vi "Overlay Landmark.vi"(6 "Color":u32(colorbox)=16711680, 7 "Group":string, 8 "error in":errorcluster, 9 "Bounding Box":cluster{"x":dbl, "y":dbl}[](array[cluster]), 10 "Position":cluster{"x":sgl, "y":sgl}, 11 "Image":T1) -> (0 "error out":errorcluster, 3 "Image Out":T1)   [LabVIEW 2024]
uses:
  <vilib>/vision/Image Controls.llb/IMAQ Image.ctl
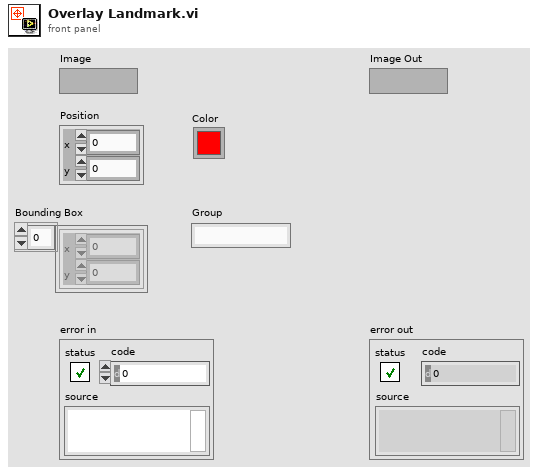
[diagram p1: front panel]
types:
  T1 = typedef "IMAQ Image.ctl" = refnum<image>
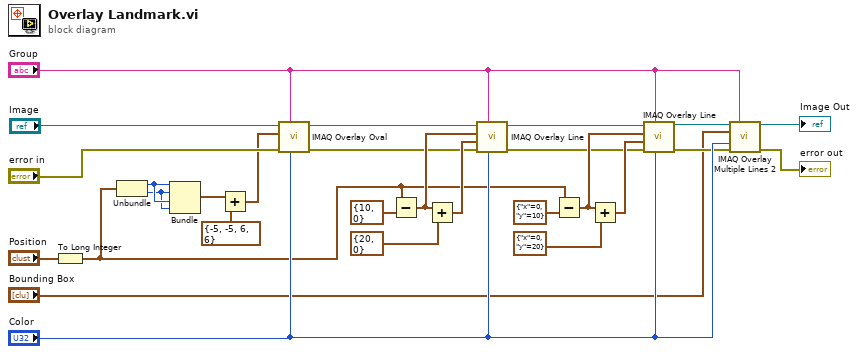
[diagram p0: block diagram]
diagram:
  n1 = To Long Integer(number="Position") -> (32bit integer=w2:cluster{"x":i32, "y":i32})
  n2 = Unbundle(w2) -> ("x"=w20:i32, "y"=w19:i32)
  n3 = Bundle("x"=w20, "y"=w19, "x"=w20, "y"=w19) -> (w18:cluster{"x":i32, "y":i32, "x":i32, "y":i32})  [unwired: 1 out]
  n4 = Add(x=w18, y=cluster{"y":i32, "x":i32, "y":i32, "x":i32} {"y"=-5, "x"=-5, "y"=6, "x"=6}) -> (x+y=w16:cluster{i32, i32, i32, i32})
  n5 = call "IMAQ Overlay Oval"("Color"="Color", "Group"="Group", "error in (no error)"="error in", "Bounding Rectangle"=w16, "Image"="Image") -> ("error out"=w6:errorcluster, "Image Out"=w22:T1)  [unwired: 1 in, 4 out]
  n6 = Subtract(x=w2, y=cluster{"x":i32, "y":i32} {"x"=10, "y"=0}) -> (x-y=w14:cluster{"x":i32, "y":i32})
  n7 = Add(x=w14, y=cluster{"x":i32, "y":i32} {"x"=20, "y"=0}) -> (x+y=w12:cluster{"x":i32, "y":i32})
  n8 = call "IMAQ Overlay Line"("Color"="Color", "Group"="Group", "error in (no error)"=w6, "End Point"=w12, "Start Point"=w14, "Image"=w22) -> ("error out"=w5:errorcluster, "Image Out"=w7:T1)  [unwired: 4 out]
  n9 = Subtract(x=w2, y=cluster{"x":i32, "y":i32} {"x"=0, "y"=10}) -> (x-y=w10:cluster{"x":i32, "y":i32})
  n10 = Add(x=w10, y=cluster{"x":i32, "y":i32} {"x"=0, "y"=20}) -> (x+y=w11:cluster{"x":i32, "y":i32})
  n11 = call "IMAQ Overlay Line"("Color"="Color", "Group"="Group", "error in (no error)"=w5, "End Point"=w11, "Start Point"=w10, "Image"=w7) -> ("error out"=w4:errorcluster, "Image Out"=w21:T1)  [unwired: 4 out]
  n12 = call "IMAQ Overlay Multiple Lines 2"("Image"=w21, "Group"="Group", "Line End Points"="Bounding Box", "Color"="Color", "error in (no error)"=w4) -> ("Image Out"=→"Image Out":T1, "error out"=→"error out":errorcluster)  [unwired: 9 in]
